vi "subvi_load_data_matrix.vi"(11 "default name":path) -> (2 "array":dbl[][](array[numeric]))   [LabVIEW 2020]
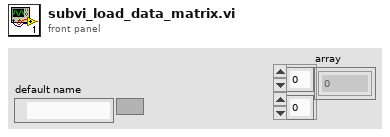
[diagram p1: front panel]
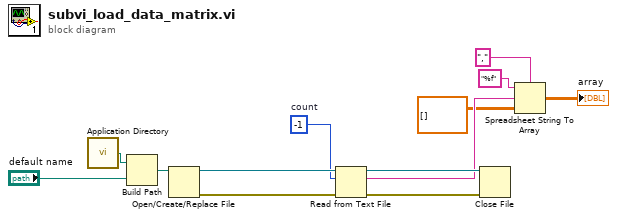
[diagram p0: block diagram]
diagram:
  w3 = -1  # count
  n1 = call <vilib>:"Application Directory.vi"() -> ("Application Directory"=w7:path)
  n2 = Build Path(base path=w7, name or relative path="default name") -> (appended path=w6:path)
  n3 = Open/Create/Replace File(file path (use dialog)=w6) -> (refnum out=w11:refnum<file>, error out=w12:errorcluster)  [unwired: 5 in, 1 out]
  n4 = Read from Text File(file (use dialog)=w11, count=w3, error in=w12) -> (refnum out=w10:refnum<file>, text=w8:string, error out=w9:errorcluster)  [unwired: 1 in, 1 out]
  n5 = Close File(refnum=w10, error in=w9) -> ()  [unwired: 2 out]
  n6 = Spreadsheet String To Array(delimiter (Tab)=",", format string="%f", spreadsheet string=w8, array type (2D Dbl)=dbl[][] []) -> (array=→"array":dbl[][])
